vi "Detect Ramp End.vi"(11 "y angle":dbl) -> (3 "Ramp Just Ended":bool)   [LabVIEW 2017]
panel:
  out "On Ramp Downside":bool
  # "There's a red line before the ramp starts,\nbut there's nothing after it ends.\n\nSo we use the gyro's y angle to figure out\nif we've finished the ramp."
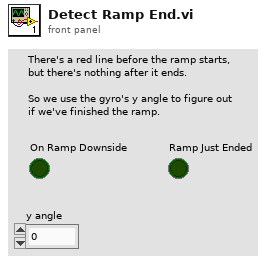
[diagram p1: front panel]
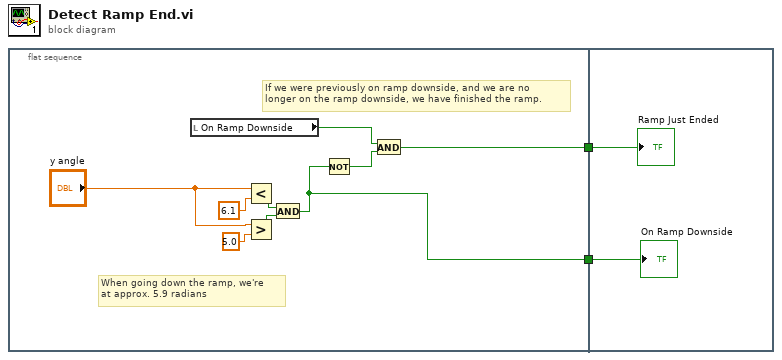
[diagram p0: block diagram]
diagram:
  n1 = flat-sequence {
    tunnel: [w3] -> w2
    tunnel: [w8] -> w1
    tunnel: w2 -> [w13]
    tunnel: w1 -> [w12]
    frame #0 {
      # "If we were previously on ramp downside, and we are no\nlonger on the ramp downside, we have finished the ramp."
      # "When going down the ramp, we're\nat approx. 5.9 radians"
      n2 = local read "On Ramp Downside"() -> (w10:bool)
      n3 = Less?(x="y angle", y=6.1) -> (x < y?=w4:bool)
      n4 = Greater?(x="y angle", y=5.0) -> (0:w5:bool)
      n5 = And(x=w4, y=w5) -> (x .and. y?=w3:bool)
      n6 = Not(x=w3) -> (.not. x?=w9:bool)
      n7 = And(x=w10, y=w9) -> (x .and. y?=w8:bool)
    }
    frame #1 {
      "On Ramp Downside" <- w13
      "Ramp Just Ended" <- w12
    }
  }
